vi "PYTHON Get Boolean Data__ogtk.vi"(4 "error in (no error)":errorcluster, 5 "data type":bool, 6 "variable name":string, 7 "Python Session in":T1) -> (0 "error out":errorcluster, 1 "value":bool, 3 "Python Session out":T1)   [LabVIEW 2014]
uses:
  <userlib>/_OpenG.lib/labpython/labpython.llb/PYTHON Session Refnum__ogtk.ctl
  <userlib>/_OpenG.lib/labpython/lvpython.dll
panel:
  # "PYTHON Get Boolean Data.vi\n\nGet the value of a boolean variable from the session context\n\nCopyright (C) 2002 Rolf Kalbermatter rolf.kalbermatter@citeng.com\nCopyright (C) 2002 James Kring jim@jimkring.com\n\nPlease visit http://www.OpenG.org to learn about the\nOpen Source LabVIEW software movement.\n\nThis library is free software; you can redistribute it and/or\nmodify it under the terms of the GNU Lesser General Public\nLicense as published by the Free Software Foundation; either\nversion 2.1 of the License, or (at your option) any later version.\nThis library is distributed in the hope that it will be useful,\nbut WITHOUT ANY WARRANTY; without even the implied warranty of\nMERCHANTABILITY or FITNESS FOR A PARTICULAR PURPOSE. See the GNU\nLesser General Public License for more details.\nYou should have received a copy of the GNU Lesser General Public\nLicense along with this library; if not, write to the Free Software\nFoundation, Inc., 59 Temple Place, Suite 330, Boston, MA 02111-1307 USA"
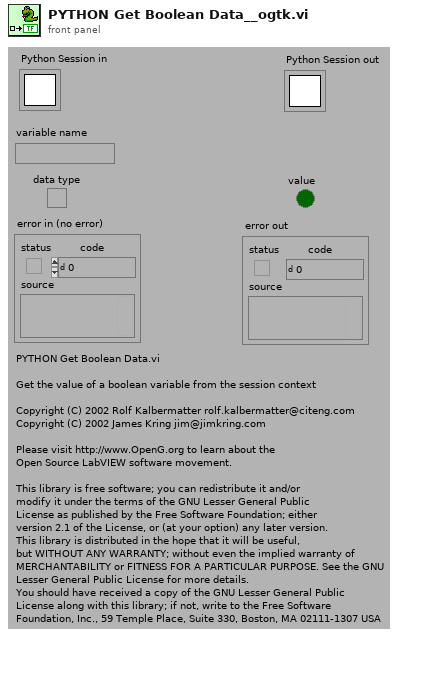
[diagram p1: front panel]
types:
  T1 = typedef "PYTHON Session Refnum__ogtk.ctl" = refnum<k1>
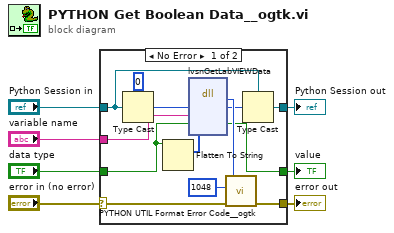
[diagram p0: block diagram]
diagram:
  n1 = case shown="No Error" "error in (no error)" {
    selector: "error in (no error)" -> [w17 w23]
    tunnel: [w9 w22] -> w1
    tunnel: [w15 w23] -> w6
    tunnel: "Python Session in" -> [w8 w22]
    tunnel: "variable name" -> [w20 _]
    tunnel: "data type" -> [w13 w21]
    tunnel: [w18 w21] -> w4
    frame No Error {
      n2 = Type Cast(type=u32 0 ("session"), x=w8) -> (*(type *) &x=w11:u32)
      n3 = Flatten To String(anything=w13) -> (type string=w14:i16[])  [unwired: 3 in, 2 out]
      n4 = dll-call lib="C:/Program Files (x86)/National Instruments/LabVIEW 2014/user.lib/_OpenG.lib/labpython/lvpython.*" fn="lvsnGetLabVIEWData"("session"=w11, "name"=w20, "data type"=w13, "type"=w14) -> (w19:i32, "session"=w10:u32, "data type"=w18:bool)  [unwired: 5 in, 2 out]
      n5 = call <userlib>:"PYTHON UTIL Format Error Code__ogtk.vi"("error in (no error)"=w17, "code"=1048, "Bool32"=w19) -> ("error out"=w15:errorcluster)  [unwired: 4 in]
      n6 = Type Cast(type=w8, x=w10) -> (*(type *) &x=w9:T1)
    }
    frame Error {
    }
  }
  "error out" <- w6
  "value" <- w4
  "Python Session out" <- w1
